vi "WaypointAndObstaclesPaint 4.vi"(11 "Sim Path":path) -> (0 "Sim Course":picture, 3 "?":u8[][](array[numeric]))   [LabVIEW 2014]
panel:
  # "Waypoint and Obstacles Paint 4"
  # "Outputs:"
  # "Input:"
  # "Inputs:"
  # "Outputs:"
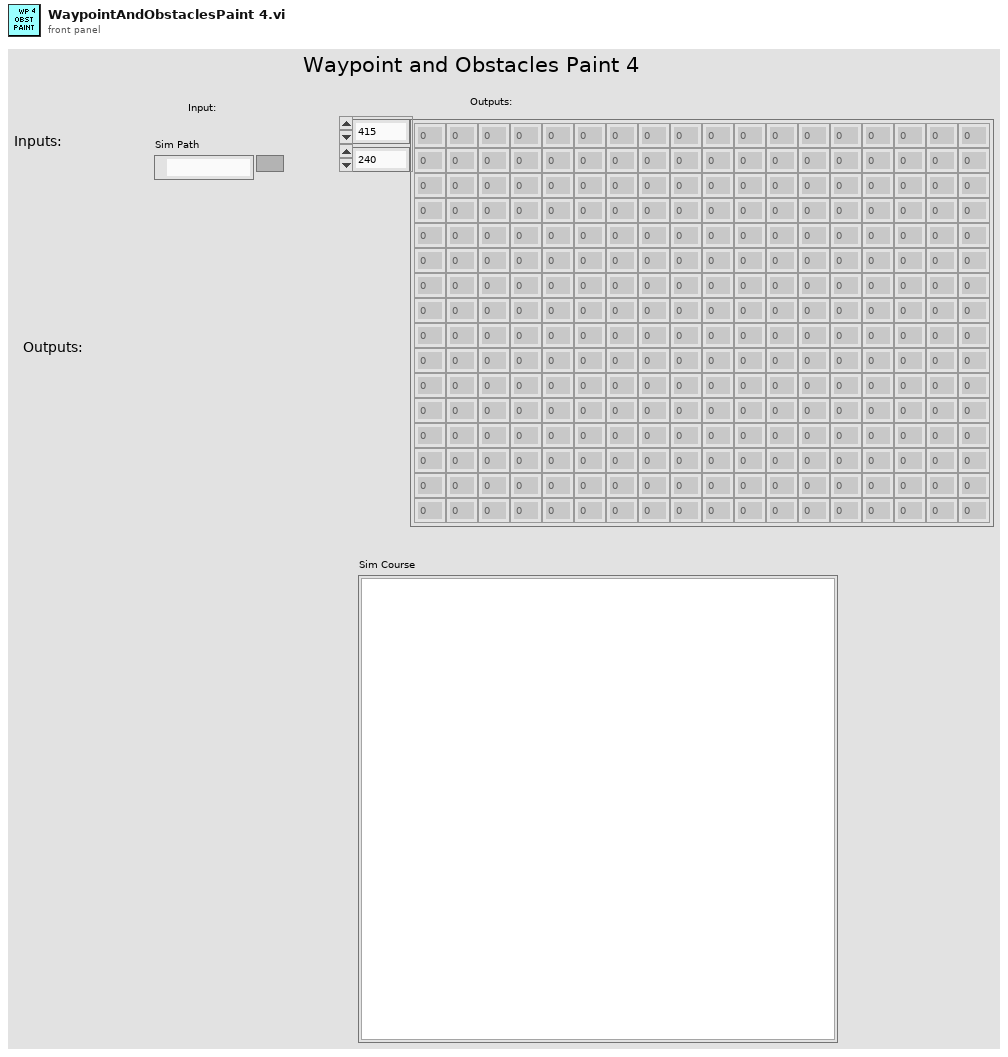
[diagram p1: front panel]
types:
  T1 = typedef "imagedata.ctl" = cluster{"image type":i32, "image depth":i32, "image":u8[], "mask":u8[], "colors":u32[], "Rectangle":cluster{"left":i16, "top":i16, "right":i16, "bottom":i16}}
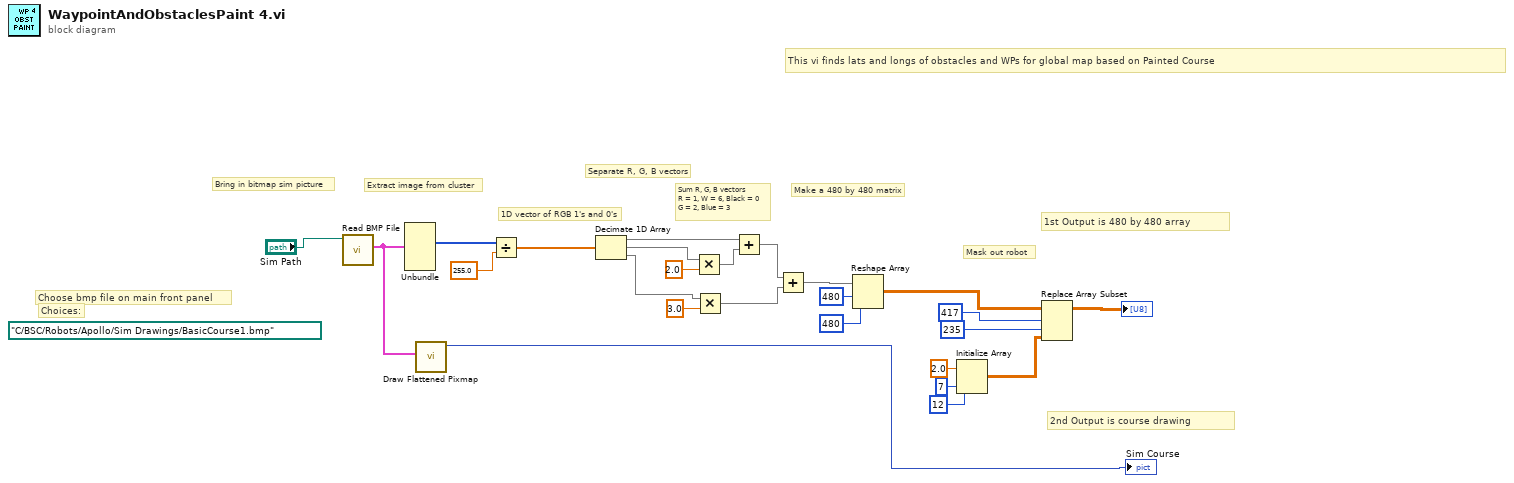
[diagram p0: block diagram]
diagram:
  (unwired) path "C:/BSC/Robots/Apollo/Sim Drawings/BasicCourse1.bmp" ("path to BMP file")
  # "Choices:"
  # "Choose bmp file on main front panel"
  # "2nd Output is course drawing"
  # "1st Output is 480 by 480 array"
  # "Mask out robot"
  # "Make a 480 by 480 matrix"
  # "Sum R, G, B vectors\nR = 1, W = 6, Black = 0\nG = 2, Blue = 3"
  # "1D vector of RGB 1's and 0's"
  # "This vi finds lats and longs of obstacles and WPs for global map based on Painted Course"
  # "Separate R, G, B vectors"
  # "Extract image from cluster"
  # "Bring in bitmap sim picture"
  n1 = call <vilib>:"Read BMP File.vi"("path to BMP file"="Sim Path") -> ("image data"=w3:T1)  [unwired: 8 in, 2 out]
  n2 = Unbundle(w3) -> ("image"=w24:u8[])  [unwired: 5 out]
  n3 = call <vilib>:"Draw Flattened Pixmap.vi"("image data"=w3) -> ("new picture"=→"Sim Course":picture)  [unwired: 8 in]
  n4 = Divide(x=w24, y=255.0) -> (x/y=w23:dbl[])
  n5 = Decimate 1D Array(w23) -> (w15:dbl[], w21:dbl[], w19:dbl[])
  n6 = Multiply(x=w21, y=2.0) -> (x*y=w18:dbl[])
  n7 = Multiply(x=w19, y=3.0) -> (x*y=w16:dbl[])
  n8 = Add(x=w15, y=w18) -> (x+y=w17:dbl[])
  n9 = Add(x=w17, y=w16) -> (x+y=w14:dbl[])
  n10 = Reshape Array(w14, 480 ("dimension size"), 480 ("dimension size")) -> (w6:dbl[][])
  n11 = Initialize Array(2.0 ("element"), 7 ("dimension size"), 12 ("dimension size")) -> (w5:dbl[][])
  n12 = Replace Array Subset(array=w6, new element=w5, index (row)=417, index (col)=235) -> (→"?":dbl[][])
